vi "Untitled 2.vi"   [LabVIEW 2020]
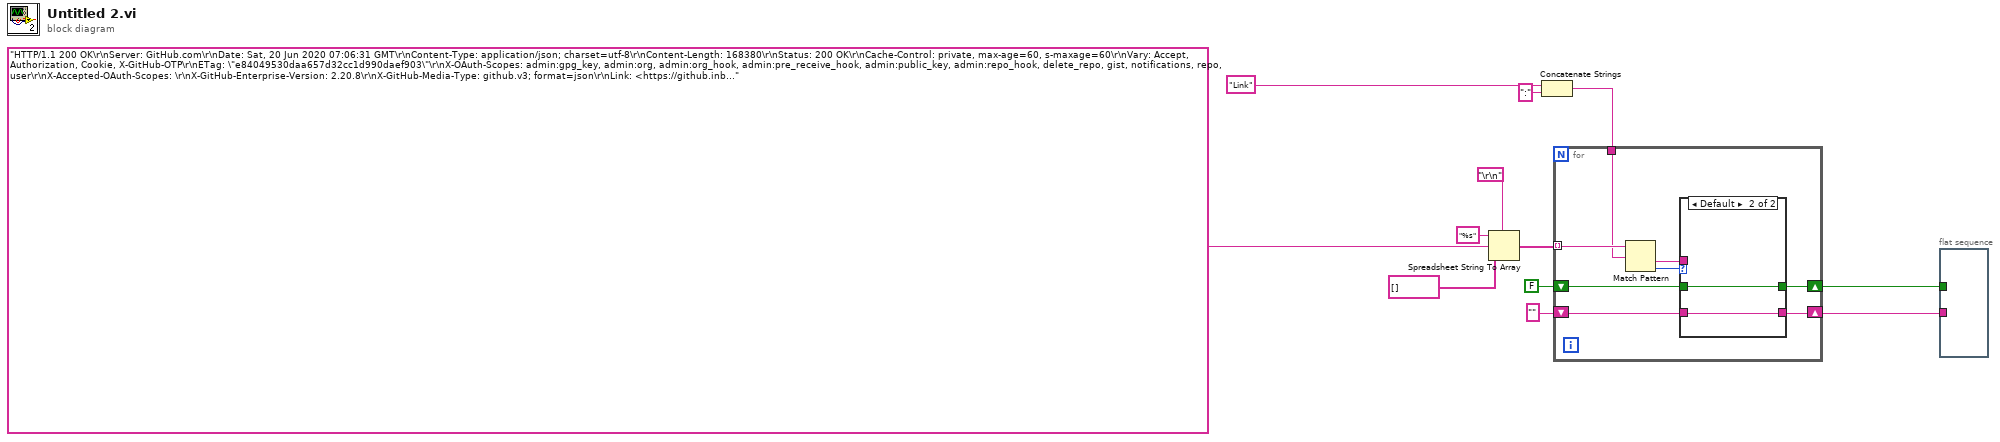
[diagram p0: block diagram]
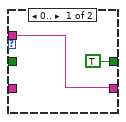
[diagram p2: hidden frame]
diagram:
  n1 = Spreadsheet String To Array(delimiter (Tab)="\r\n", format string="%s", spreadsheet string="HTTP/1.1 200 OK\r\nServer: GitHub.com\r\nDate: Sat, 20 Jun 2020 07:06:31 GMT\r\nContent-Type: application/json; charset=utf-8\r\nContent-Length: 168380\r\nStatus: 200 OK\r\nCache-Control: private, max-age=60, s-maxage=60\r\nVary: Accept, Authorization, Cookie, X-GitHub-OTP\r\nETag: \"e84049530daa657d32cc1d990daef903\"\r\nX-OAuth-Scopes: admin:gpg_key, admin:org, admin:org_hook, admin:pre_receive_hook, admin:public_key, admin:repo_hook, delete_repo, gist, notifications, repo, user\r\nX-Accepted-OAuth-Scopes: \r\nX-GitHub-Enterprise-Version: 2.20.8\r\nX-GitHub-Media-Type: github.v3; format=json\r\nLink: <https://github.inbcu.com/api/v3/organizations/1035/repos?page=2>; rel=\"next\", <https://github.inbcu.com/api/v3/organizations/1035/repos?page=6>; rel=\"last\"\r\nAccess-Control-Expose-Headers: ETag, Link, Location, Retry-After, X-GitHub-OTP, X-RateLimit-Limit, X-RateLimit-Remaining, X-RateLimit-Reset, X-OAuth-Scopes, X-Accepted-OAuth-Scopes, X-Poll-Interval, X-GitHub-Media-Type\r\nAccess-Control-Allow-Origin: *\r\nX-GitHub-Request-Id: e46bbbd4-af6d-45b2-9a2d-4b9ce20a30f7\r\nStrict-Transport-Security: max-age=31536000; includeSubdomains\r\nX-Frame-Options: deny\r\nX-Content-Type-Options: nosniff\r\nX-XSS-Protection: 1; mode=block\r\nReferrer-Policy: origin-when-cross-origin, strict-origin-when-cross-origin\r\nContent-Security-Policy: default-src 'none'\r\nX-Runtime-rack: 0.648899\r\n\r\n", array type (2D Dbl)=string[] []) -> (array=w8:string[])
  n2 = Concatenate Strings("Link", ":" ("string")) -> (w5:string)
  n3 = for {
    tunnel: w8 -> [w20] mode=indexing
    tunnel: w5 -> [w19]
    shift-right: [w17] -> w3
    shift-left: "" ("after substring") -> [w18]
    shift-right: [w13] -> w1
    shift-left: FALSE -> [w14]
    n4 = Match Pattern(string=w20, regular expression=w19) -> (after substring=w15:string, offset past match=w16:i32)  [unwired: 1 in, 2 out]
    n5 = case shown="Default" w16 {
      tunnel: w18 -> [_ w24]
      tunnel: [w22 w24] -> w17
      tunnel: w15 -> [w22 _]
      tunnel: [TRUE w23] -> w13
      tunnel: w14 -> [_ w23]
      frame 0.. {
      }
      frame Default {
      }
    }
  }
  n6 = flat-sequence {
    tunnel: w3 -> [_]
    tunnel: w1 -> [_]
    frame #0 {
    }
  }
